vi "Recall Save Parameter Settings File.vi"(0 "VISA resource name":refnum<visa-resource-name>, 5 "Application Target Setting (0: Recall All)":i32(ring) items=["Recall All", "Recall Current", "Save"], 9 "Target Filename (TEST)":string="TEST", 11 "error in (no error)":errorcluster, 12 "Driver Letter (D)":string="D") -> (4 "VISA resource name out":refnum<visa-resource-name>, 15 "error out":errorcluster)   [LabVIEW 2020, in "Anritsu Signal Analyzer Series.lvlib"]
doc: "Restores (current or all) or Saves settings of the application to the parameter setting file contents."
uses:
  Anritsu Signal Analyzer Series.lvlib
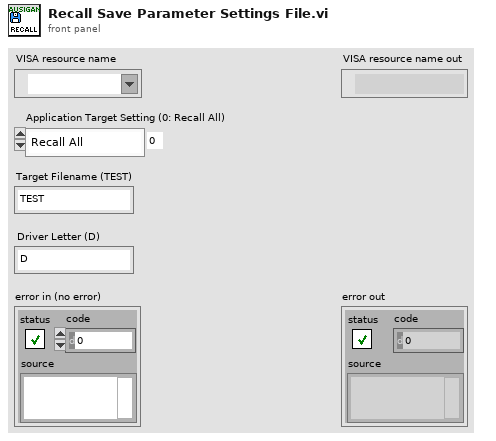
[diagram p1: front panel]
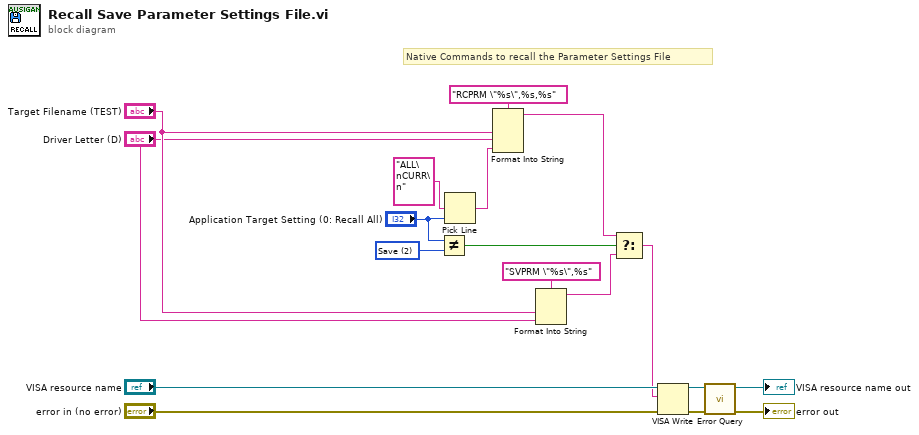
[diagram p0: block diagram]
diagram:
  w9 = 2 items=["Recall All", "Recall Current", "Save"] ("Parameter Settings Action (0:All) 2")
  # "Native Commands to recall the Parameter Settings File"
  n1 = Not Equal?(x="Application Target Setting (0: Recall All)", y=w9) -> (x != y?=w7:bool)
  n2 = Pick Line(multi-line string="ALL\nCURR\n", line index="Application Target Setting (0: Recall All)") -> (output string=w10:string)  [unwired: 1 in]
  n3 = Format Into String(format string="RCPRM \"%s\",%s,%s" ("_Command"), "Target Filename (TEST)", "Driver Letter (D)", w10) -> (resulting string=w6:string)  [unwired: 2 in, 1 out]
  n4 = Format Into String(format string="SVPRM \"%s\",%s" ("_Command"), "Target Filename (TEST)", "Driver Letter (D)") -> (resulting string=w4:string)  [unwired: 2 in, 1 out]
  n5 = Select(t=w6, s=w7, f=w4) -> (s? t:f=w1:string)
  n6 = VISA Write(VISA resource name="VISA resource name", write buffer=w1, error in (no error)="error in (no error)") -> (VISA resource name out=w12:refnum<visa-resource-name>, error out=w13:errorcluster)  [unwired: 1 out]
  n7 = call "Error Query.vi"("error in (no error)"=w13, "VISA resource name"=w12) -> ("error out"=→"error out":errorcluster, "VISA resource name out"=→"VISA resource name out":refnum<visa-resource-name>)  [unwired: 6 in, 2 out]
